vi "Get Size.vi"(8 "error in (no error)":errorcluster, 11 "Glyph Destination in":refnum<class "VI Icon Canvas.lvclass">) -> (0 "error out":errorcluster, 2 "Size":cluster{"Width":u16, "Height":u16}, 3 "Glyph Destination out":refnum<class "VI Icon Canvas.lvclass">)   [LabVIEW 2023, in "Font Glyph Drawer Interface.lvlib" / "VI Icon Canvas.lvclass"]
uses:
  VI Icon Canvas.lvclass
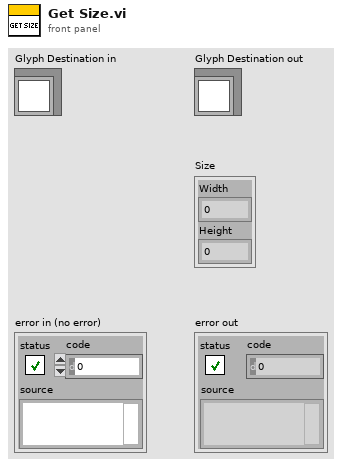
[diagram p1: front panel]
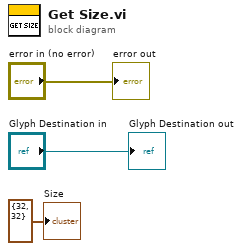
[diagram p0: block diagram]
diagram:
  "error out" <- "error in (no error)"
  "Glyph Destination out" <- "Glyph Destination in"
  "Size" <- cluster{"Width":u16, "Height":u16} {"Width"=32, "Height"=32} ("Size")
